vi "Profile scan start (SubVI).vi"(3 "error in":errorcluster, 4 "Шаг":i32, 5 "Конец области":dbl, 6 "VISA Refnum in":refnum<visa-resource-name>) -> (0 "error out":errorcluster, 1 "Profile":cluster{dbl[], dbl[]}, 2 "pos_z":dbl)   [LabVIEW 2018]
uses:
  GlobalStop.vi
panel:
  out "str_array":string[][](array[string])
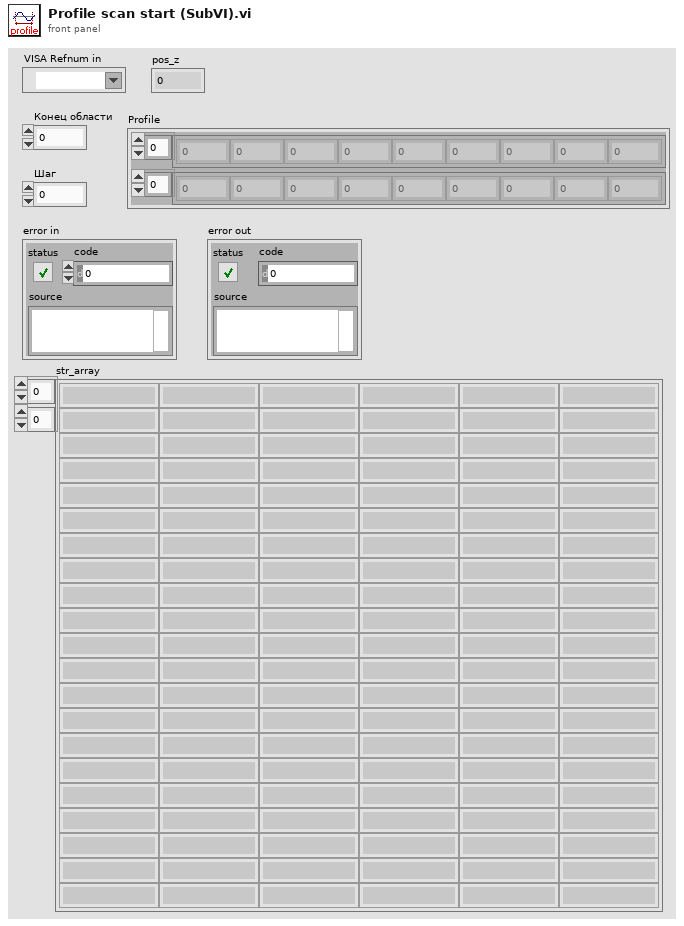
[diagram p1: front panel]
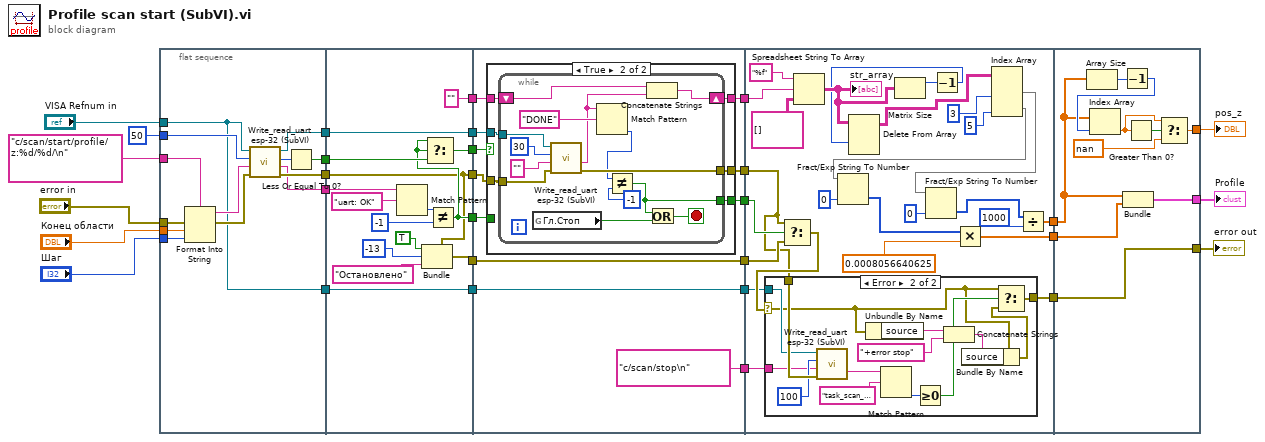
[diagram p0: block diagram]
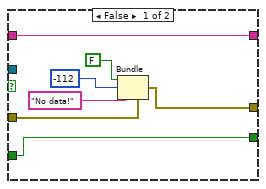
[diagram p2: hidden frame]
diagram:
  n1 = flat-sequence {
    tunnel: "Шаг" -> [w42]
    tunnel: "Конец области" -> [w41]
    tunnel: "error in" -> [w39]
    tunnel: "c/scan/start/profile/z:%d/%d/\n" ("format string") -> [w38]
    tunnel: u32 50 ("milliseconds to wait") -> [w36]
    tunnel: "VISA Refnum in" -> [w31]
    tunnel: [w43] -> w24
    tunnel: [w34] -> w23
    tunnel: [w33] -> w22
    tunnel: [w32] -> w21
    tunnel: [w31] -> w3
    tunnel: w24 -> [w48]
    tunnel: w23 -> [w53]
    tunnel: w22 -> [w54]
    tunnel: w21 -> [w55]
    tunnel: [w48] -> w20
    tunnel: [w51] -> w19
    tunnel: [w54] -> w18
    tunnel: [w52] -> w17
    tunnel: [""] -> w16
    tunnel: [w46] -> w11
    tunnel: [w45] -> w4
    tunnel: w3 -> [w45]
    tunnel: w20 -> [w67]
    tunnel: w19 -> [w66]
    tunnel: w18 -> [w69]
    tunnel: w17 -> [w68]
    tunnel: w16 -> [w65]
    tunnel: [w64] -> w15
    tunnel: [w63] -> w14
    tunnel: [w62] -> w13
    tunnel: [w61] -> w12
    tunnel: w11 -> [w61]
    tunnel: [w60] -> w5
    tunnel: w4 -> [w60]
    tunnel: ["c/scan/stop\n" ("format string")] -> w2
    tunnel: w15 -> [w121]
    tunnel: w14 -> [w111]
    tunnel: w13 -> [w98]
    tunnel: w12 -> [w100]
    tunnel: [w110] -> w10
    tunnel: [w108] -> w9
    tunnel: w5 -> [w101]
    tunnel: w2 -> [w99]
    tunnel: [w97] -> w1
    tunnel: w10 -> [w139]
    tunnel: w9 -> [w140]
    tunnel: [w142] -> w8
    tunnel: [w141] -> w7
    tunnel: [w138] -> w6
    tunnel: w1 -> [w142]
    frame #0 {
      n2 = Format Into String(format string=w38, error in=w39, w41, w42) -> (resulting string=w37:string, error out=w40:errorcluster)  [unwired: 1 in]
      n3 = call "Write_read_uart esp-32 (SubVI).vi"("error in (no error)"=w40, "write buffer"=w37, "milliseconds to wait"=w36, "VISA Refnum in"=w31) -> ("error out 4"=w43:errorcluster, "read buffer"=w32:string, "read bite"=w35:u32, "VISA resource name out"=w33:refnum<visa-resource-name>)
      n4 = Less Or Equal To 0?(x=w35) -> (x <= 0?=w34:bool)
    }
    frame #1 {
      n5 = Match Pattern(string=w55, regular expression="uart: OK") -> (offset past match=w56:i32)  [unwired: 1 in, 3 out]
      n6 = Bundle(cluster=w48, "status"=TRUE, "code"=-13, "source"="Остановлено") -> (w46:errorcluster)
      n7 = Not Equal?(x=w56, y=-1 ("offset past match")) -> (x != y?=w51:bool)
      n8 = Select(t=w51, s=w51, f=w53) -> (s? t:f=w52:bool)
    }
    frame #2 {
      n9 = case shown="True" w68 {
        tunnel: w67 -> [w74 w82]
        tunnel: w69 -> [_ w81]
        tunnel: [w70 w80] -> w62
        tunnel: [w76 w79] -> w63
        tunnel: w66 -> [w76 _]
        tunnel: w65 -> [w75 w78]
        tunnel: [w75 w77] -> w64
        frame False {
          n10 = Bundle(cluster=w74, "status"=FALSE, "code"=-112, "source"="No data!") -> (w70:errorcluster)
        }
        frame True {
          n11 = while {
            tunnel: w82 -> [w94]
            tunnel: w81 -> [w93]
            tunnel: [w89] -> w80
            tunnel: [w87] -> w79
            shift-right: [w84] -> w77
            shift-left: w78 -> [w85]
            stop <- w90 stop-if-true
            n12 = global read "GlobalStop.vi" "Гл.Стоп"() -> (w86:bool)
            n13 = call "Write_read_uart esp-32 (SubVI).vi"("error in (no error)"=w94, "write buffer"="", "milliseconds to wait"=u32 30, "VISA Refnum in"=w93) -> ("error out 4"=w89:errorcluster, "read buffer"=w83:string)  [unwired: 2 out]
            n14 = Match Pattern(string=w83, regular expression="DONE") -> (offset past match=w88:i32)  [unwired: 1 in, 3 out]
            n15 = Not Equal?(x=w88, y=-1 ("offset past match")) -> (x != y?=w87:bool)
            n16 = Concatenate Strings(w85, w83) -> (w84:string)
            n17 = Or(x=w87, y=w86) -> (x .or. y?=w90:bool)
          }
        }
      }
    }
    frame #3 {
      n18 = Select(t=w98, s=w111, f=w100) -> (s? t:f=w102:errorcluster)
      n19 = case shown="Error" w102 {
        selector: w102 -> [w123 w129]
        tunnel: w101 -> [_ w130]
        tunnel: w98 -> [_ w137]
        tunnel: w99 -> [_ w135]
        tunnel: [w123 w124] -> w97
        frame No Error {
        }
        frame Error {
          n20 = call "Write_read_uart esp-32 (SubVI).vi"("error in (no error)"=w137, "write buffer"=w135, "milliseconds to wait"=u32 100, "VISA Refnum in"=w130) -> ("read buffer"=w134:string)  [unwired: 3 out]
          n21 = Unbundle By Name(w129) -> ("source"=w128:string)
          n22 = Match Pattern(string=w134, regular expression="task_scan_pp - STOP") -> (offset past match=w132:i32)  [unwired: 1 in, 3 out]
          n23 = Greater Or Equal To 0?(x=w132) -> (x >= 0?=w131:bool)
          n24 = Concatenate Strings(w128, "+error stop") -> (w126:string)
          n25 = Bundle By Name(cluster=w129, "source"=w126) -> (w127:errorcluster)
          n26 = Select(t=w129, s=w131, f=w127) -> (s? t:f=w124:errorcluster)
        }
      }
      n27 = Spreadsheet String To Array(format string="%f", spreadsheet string=w121, array type (2D Dbl)=string[][] [] ("Array")) -> (array=w106:string[][])  [unwired: 1 in]
      "str_array" <- w106
      n28 = Matrix Size(0:w106) -> (1:w107:i32)  [unwired: 1 out]
      n29 = Decrement(x=w107) -> (x-1=w105:i32)
      n30 = Delete From Array(array=w106, index (row)=w105) -> (array with subset deleted=w104:string[][])  [unwired: 2 in, 1 out]
      n31 = Index Array(array=w104, index (col) #1=3 ("index (row)"), index (col) #2=5 ("index (col)")) -> (element #1=w114:string[], element #2=w116:string[])  [unwired: 2 in]
      n32 = Fract/Exp String To Number(string=w116, default (0 dbl)=i16 0 ("default (0 DBL)")) -> (number=w112:i16[])  [unwired: 3 out]
      n33 = Fract/Exp String To Number(string=w114, default (0 dbl)=i16 0 ("default (0 DBL)")) -> (number=w103:i16[])  [unwired: 3 out]
      n34 = Multiply(x=w112, y=0.0008056640625) -> (x*y=w110:dbl[])
      n35 = Divide(x=w103, y=1000) -> (x/y=w108:dbl[])
    }
    frame #4 {
      n36 = Array Size(array=w140) -> (size(s)=w147:i32)
      n37 = Decrement(x=w147) -> (x-1=w146:i32)
      n38 = Index Array(array=w140, index=w146) -> (element=w144:dbl)
      n39 = Bundle(w140, w139) -> (w138:cluster{dbl[], dbl[]})  [unwired: 1 in]
      n40 = Greater Than 0?(x=w144) -> (x > 0?=w145:bool)
      n41 = Select(t=w144, s=w145, f=nan) -> (s? t:f=w141:dbl)
    }
  }
  "error out" <- w8
  "pos_z" <- w7
  "Profile" <- w6
